vi "Test 4.vi"(8 "error in (no error)":errorcluster, 11 "Test Case In":refnum<class "Tests.lvclass">) -> (0 "error out":errorcluster, 3 "Test Case Out":refnum<class "Tests.lvclass">)   [LabVIEW 2020, in "Tests.lvclass"]
uses:
  Tests.lvclass
  C:/Program Files (x86)/National Instruments/LabVIEW 2020/vi.lib/Astemes/LUnit/Test Case.lvclass
  <vilib>/Astemes/LUnit/Test Case.lvclass/Test Case.ctl
  4993e8ee-a06a-463a-9684-69129f64d5ce.vi
  <vilib>/Astemes/LUnit/Append Pass Result.vi
  <vilib>/Astemes/LUnit/Append Fail Result.vi
  <vilib>/Astemes/LUnit/Describe Comparison.vi
  4993e8ee-a06a-463a-9684-69129f64d5ce.vi/9c5d11cd-9439-4240-a1ee-d9baace9c924.vi
  <vilib>/Astemes/LUnit/Run In UI.vi
  <vilib>/Utility/error.llb/Clear Errors.vi
  <vilib>/Astemes/LUnit/Describe Variant.vi
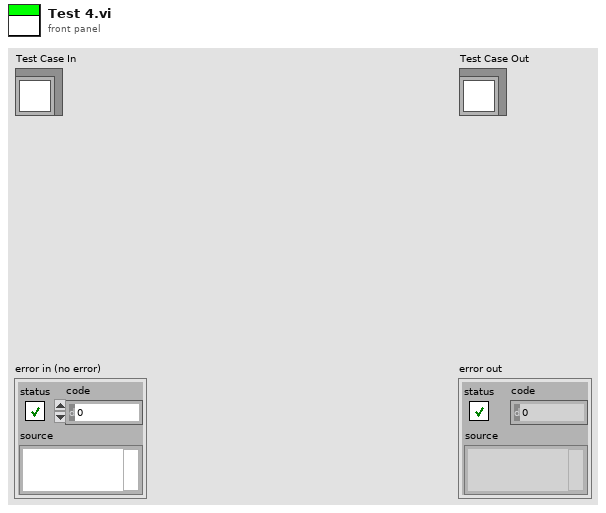
[diagram p1: front panel]
types:
  T1 = cluster{cluster{"String":string, "String":string}, cluster{"String":string, "String":string}}[]
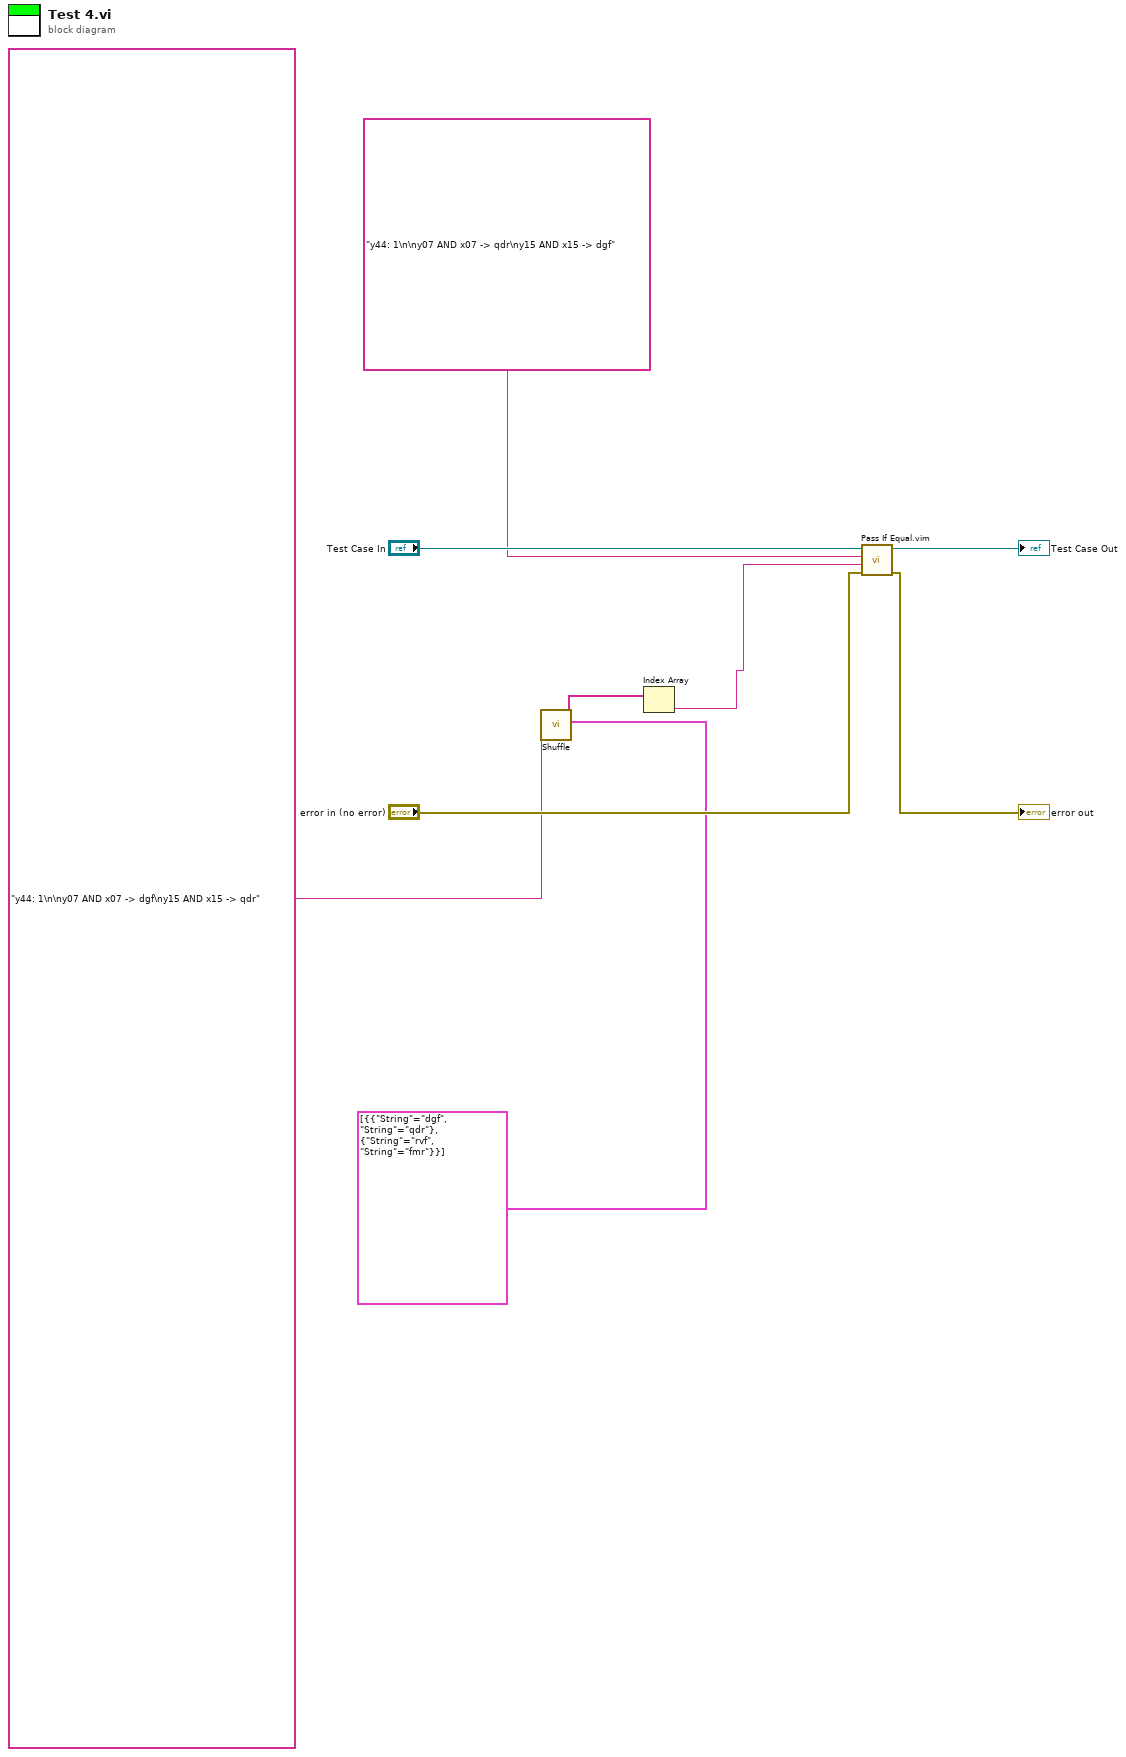
[diagram p0: block diagram]
diagram:
  n1 = call "Shuffle.vi"("Array in"=T1 [{{"String"="dgf", "String"="qdr"}, {"String"="rvf", "String"="fmr"}}], "Input"="y44: 1\n\ny07 AND x07 -> dgf\ny15 AND x15 -> qdr") -> ("Array out"=w3:string[])  [unwired: 9 in]
  n2 = Index Array(array=w3) -> (element=w2:string)  [unwired: 1 in]
  n3 = call "Pass If Equal.vim"("error in (no error)"="error in (no error)", "Actual"=w2, "Expected"="y44: 1\n\ny07 AND x07 -> qdr\ny15 AND x15 -> dgf" ("Input"), "LUnit Test Case In"="Test Case In") -> ("error out"=→"error out":errorcluster, "LUnit Test Case Out"=→"Test Case Out":refnum<class "Tests.lvclass">)  [unwired: 6 in]
